vi "Write Parent.vi"(8 "Error In":errorcluster, 10 "Parent":refnum<class "Abstract.lvclass">, 11 "Node In":refnum<class "Terminal.lvclass">) -> (0 "Error Out":errorcluster, 3 "Node Out":refnum<class "Terminal.lvclass">)   [LabVIEW 2018, in "Toolkit.lvlib" / "Nodes.lvlib" / "Terminal.lvclass"]
uses:
  Terminal.lvclass
  Abstract/Abstract.lvclass
  Terminal.lvclass/Terminal.ctl
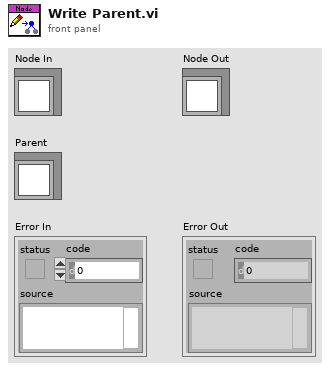
[diagram p1: front panel]
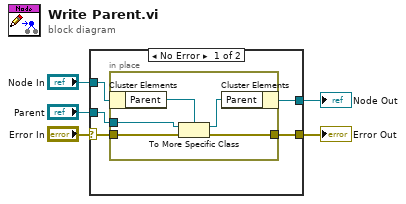
[diagram p0: block diagram]
diagram:
  n1 = case shown="No Error" "Error In" {
    selector: "Error In" -> [w7 w16]
    tunnel: "Parent" -> [w9 _]
    tunnel: "Node In" -> [w10 w17]
    tunnel: [w8 w17] -> w2
    tunnel: [w6 w16] -> w1
    frame No Error {
      n2 = in-place {
        in-place-border: w9 -> [w13]
        in-place-border: w7 -> [w15]
        in-place-border: [w14] -> w6
        n3 = in-place-cluster #1(w10) -> ("Parent"=w12:refnum<class "NonTerminal.lvclass">)
        n4 = To More Specific Class(target class=w12, reference=w13, error in=w15) -> (specific class reference=w11:refnum<class "NonTerminal.lvclass">, error out=w14:errorcluster)
        n5 = in-place-cluster #1("Parent"=w11) -> (w8:refnum<class "Terminal.lvclass">)
      }
    }
    frame Error {
    }
  }
  "Error Out" <- w1
  "Node Out" <- w2
